vi "Services.Compile.vi"(8 "error in (no error)":errorcluster, 11 "Section Ref in":T4 format="%.0x") -> (0 "error out":errorcluster, 2 "Settings":T1[](array[typedef]) {"Signal.Cmd.Refs"."Signal Refs" format="%.0x"; "Signal.Cmd.Info"."Signals"."Byte Order" items=["Little Endian", "Big Endian"]; "Signal.Cmd.Info"."Signals"."Data Type" items=["Signed", "Unsigned", "IEEE Float"]; "Settings.Refs"."Signal Refs" format="%.0x"; "Signal.Resp.Refs"."Signal Refs" format="%.0x"; "Signal.Resp.Info"."Signals"."Byte Order" items=["Little Endian", "Big Endian"]; "Signal.Resp.Info"."Signals"."Data Type" items=["Signed", "Unsigned", "IEEE Float"]; "Trigger.Refs"."Signal Refs" format="%.0x"; "Status.Refs"."Signal Refs" format="%.0x"}, 3 "Section Ref out":T4 format="%.0x")   [LabVIEW 2019, in "Diagnostics Addon System Explorer.lvlib"]
uses:
  Diagnostics Addon System Explorer.lvlib
  <vilib>/NI VeriStand/Custom Device Tools/Custom Device Utility Library/Custom Device Utility Library.lvlib
  Types/Frame.Ref.ctl
  Types/FG.Action.ctl
  <vilib>/NI VeriStand/Custom Device API/Custom Device Item Ref.ctl
  <vilib>/NI VeriStand/Custom Device API/Custom Device API.lvlib
  Addon Shared/Types/Signal.ctl
  Addon Shared/Diagnostics Addon Shared.lvlib
  Addon Shared/Types/Frame.Compile.ctl
  Addon Shared/Types/Type.ctl
  Types/Service.Export.ctl
  <vilib>/NI VeriStand/Custom Device Tools/Custom Device Utility Library/NI VeriStand - Search for Item by GUID.vi
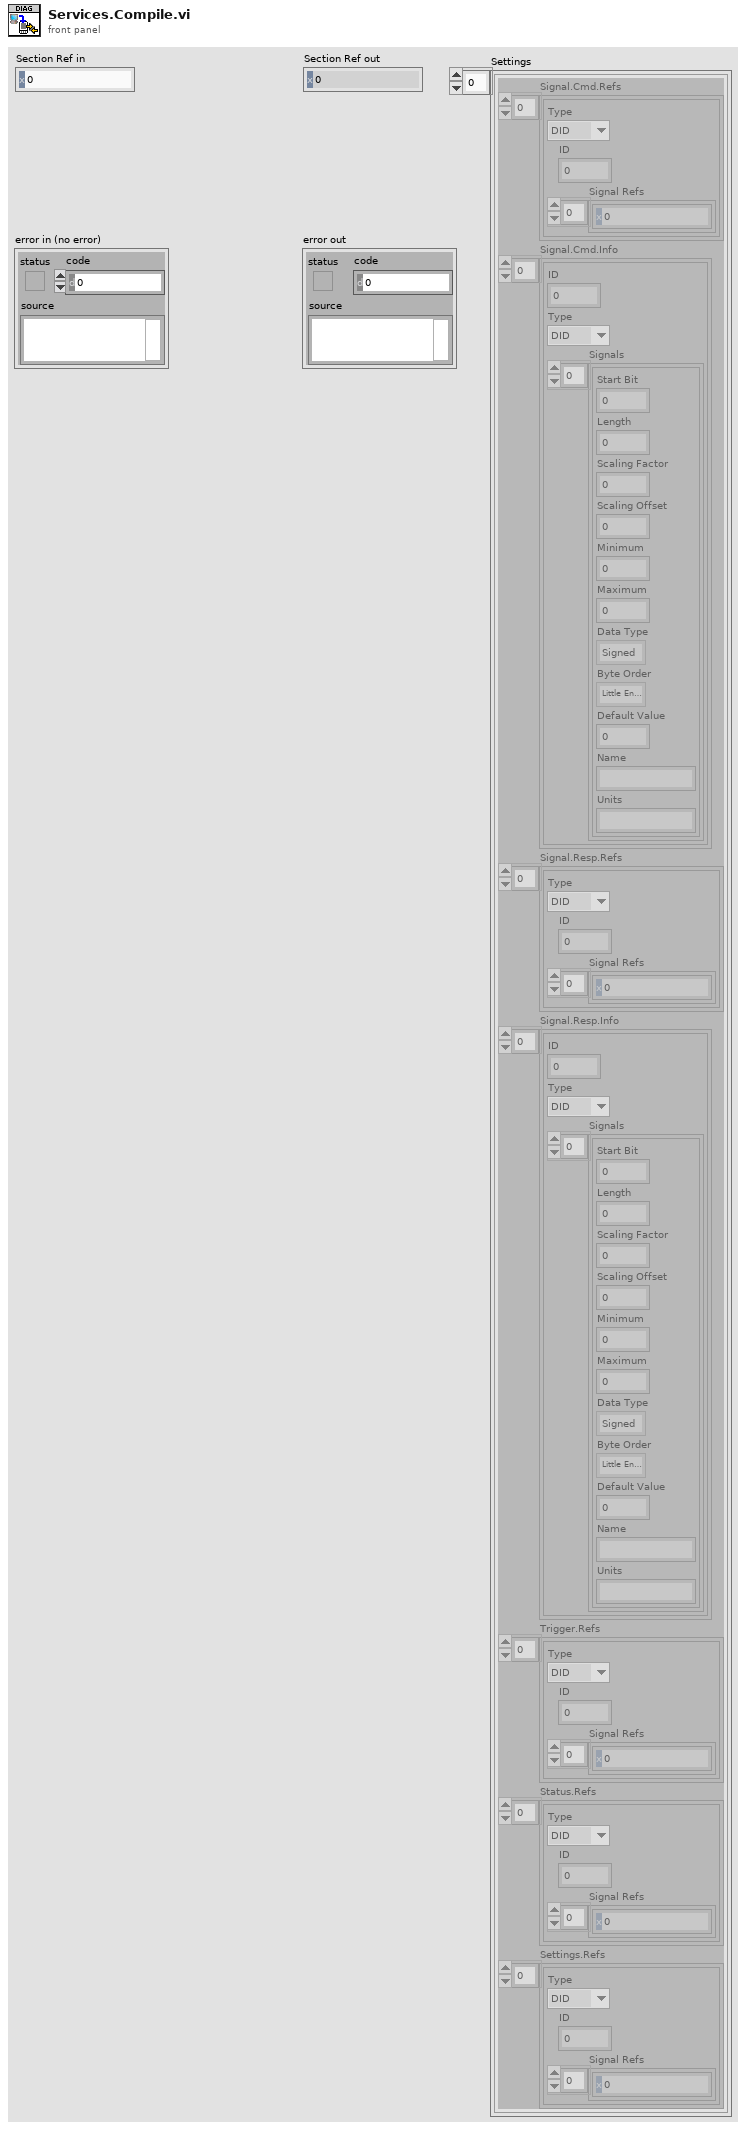
[diagram p1: front panel]
types:
  T1 = typedef "Diagnostics Addon System Explorer.lvlib/Service.Export.ctl" = cluster{"Signal.Cmd.Refs":T2[], "Signal.Cmd.Info":T5[], "Signal.Resp.Refs":T2[], "Signal.Resp.Info":T5[], "Trigger.Refs":T2[], "Status.Refs":T2[], "Settings.Refs":T2[]}
  T2 = typedef "Diagnostics Addon System Explorer.lvlib/Frame.Ref.ctl" = cluster{"Type":T3, "ID":u32, "Signal Refs":T4[]}
  T3 = typedef "Diagnostics Addon Shared.lvlib/Type.ctl" = enum16{"DID", "CDID", "PID", "CPID", "Read Memory", "Write Memory", "IO Control", "Routine Start", "Routine Request", "Routine Stop", "User Defined", "DTC Control", "Clear DTCs", "Read DTCs", "Start DTCs", "DTC Change Count", "Tester Present", "Unlock ECU", "Reset ECU", "Diag Session Control", "Communication Control", "DPID Control", "Poll Control", "Diag Comm Port Control"}
  T4 = typedef "Custom Device API.lvlib/Custom Device Item Ref.ctl" = u64
  T5 = typedef "Diagnostics Addon Shared.lvlib/Frame.Compile.ctl" = cluster{"ID":u32, "Type":T3, "Signals":T6[]}
  T6 = typedef "Diagnostics Addon Shared.lvlib/Signal.ctl" = cluster{"Start Bit":u32, "Length":u32, "Scaling Factor":dbl, "Scaling Offset":dbl, "Minimum":dbl, "Maximum":dbl, "Data Type":u32, "Byte Order":u32, "Default Value":dbl, "Name":string, "Units":string}
  T7 = typedef "Diagnostics Addon System Explorer.lvlib/FG.Action.ctl" = enum16{"Get", "Set"}
  T8 = typedef "Diagnostics Addon Shared.lvlib/CAN.ctl" = cluster{"Interface":T9, "Baud Rate":u64, "Diagnostic Protocol":T10, "Transport Protocol":T11, "Transmit ID":u32, "Receive ID":u32, "Transmit Extension":u8, "Receive Extension":u8, "Receive UUDT ID":u32, "Enable Stream":bool, "VW TP Channel ID":u32, "Fill Frame":bool, "Fill Byte":u8, "Termination":bool, "LIN Cluster":refnum<k21>, "NAD":u8, "IO Mode":u32, "Max DLC":u16, "FD Baud Rate":u64, "Timeout":u32, "FD ISO Mode":u32, "DoIP Address":string, "DoIP Source Address":u16, "DoIP Dynamic Port":bool, "DoIP Version":u16}
  T9 = typedef "Diagnostics Addon Shared.lvlib/CAN.Interface.ctl" = string
  T10 = typedef "Diagnostics Addon Shared.lvlib/Protocol.ctl" = enum16{"GMLAN", "KWP-2000", "UDS", "User-Defined"}
  T11 = typedef "Diagnostics Addon Shared.lvlib/Transport.ctl" = enum16{"ISO TP - Normal Mode", "ISO TP - Mixed Mode", "VW TP 2.0", "Diagnostics on IP", "ISO TP LIN"}
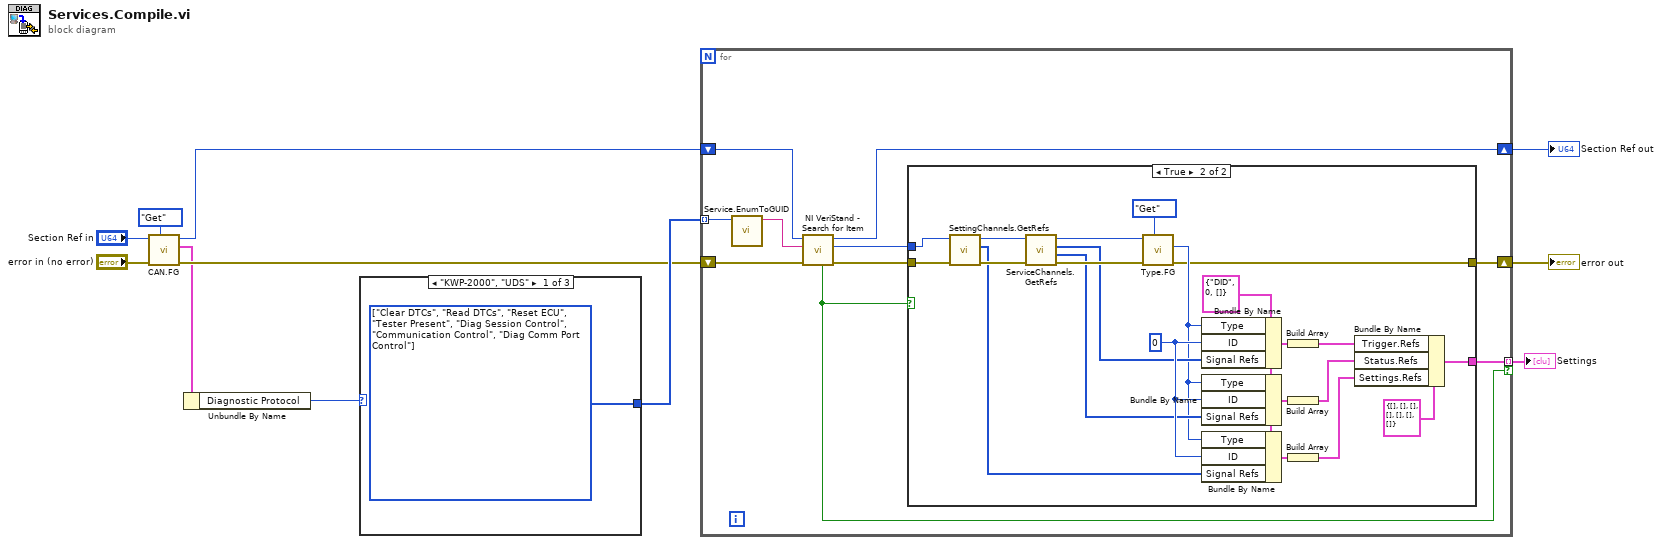
[diagram p0: block diagram]
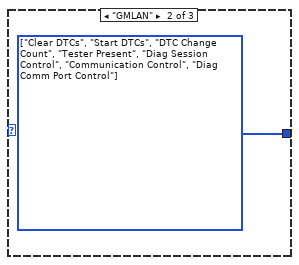
[diagram p2: hidden frame]
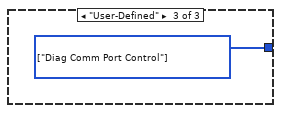
[diagram p3: hidden frame]
diagram:
  n1 = call "CAN.FG.vi"("Action"=FG.Action."Get", "error in (no error)"="error in (no error)", "Device Item Ref in"="Section Ref in") -> ("error out"=w5:errorcluster, "Diagnostics Basic Configuration"=w2:T8, "Device Item Ref out"=w3:T4)  [unwired: 6 in]
  n2 = Unbundle By Name(w2) -> ("Diagnostic Protocol"=w1:T10)
  n3 = case shown="\"KWP-2000\", \"UDS\"" w1 {
    tunnel: [w12 w13 w14] -> w8
    frame "KWP-2000", "UDS" {
      w12 = T3[] [enum."Clear DTCs", enum."Read DTCs", enum."Reset ECU", enum."Tester Present", enum."Diag Session Control", enum."Communication Control", enum."Diag Comm Port Control"] items=["DID", "CDID", "PID", "CPID", "Read Memory", "Write Memory", "IO Control", "Routine Start", "Routine Request", "Routine Stop", "User Defined", "DTC Control", "Clear DTCs", "Read DTCs", "Start DTCs", "DTC Change Count", "Tester Present", "Unlock ECU", "Reset ECU", "Diag Session Control", "Communication Control", "DPID Control", "Poll Control", "Diag Comm Port Control"]
    }
    frame "GMLAN" {
      w13 = T3[] [enum."Clear DTCs", enum."Start DTCs", enum."DTC Change Count", enum."Tester Present", enum."Diag Session Control", enum."Communication Control", enum."Diag Comm Port Control"] items=["DID", "CDID", "PID", "CPID", "Read Memory", "Write Memory", "IO Control", "Routine Start", "Routine Request", "Routine Stop", "User Defined", "DTC Control", "Clear DTCs", "Read DTCs", "Start DTCs", "DTC Change Count", "Tester Present", "Unlock ECU", "Reset ECU", "Diag Session Control", "Communication Control", "DPID Control", "Poll Control", "Diag Comm Port Control"]
    }
    frame "User-Defined" {
      w14 = T3[] [enum."Diag Comm Port Control"] items=["DID", "CDID", "PID", "CPID", "Read Memory", "Write Memory", "IO Control", "Routine Start", "Routine Request", "Routine Stop", "User Defined", "DTC Control", "Clear DTCs", "Read DTCs", "Start DTCs", "DTC Change Count", "Tester Present", "Unlock ECU", "Reset ECU", "Diag Session Control", "Communication Control", "DPID Control", "Poll Control", "Diag Comm Port Control"]
    }
  }
  n4 = for {
    tunnel: [w18] -> w9 mode=indexing if=w17
    shift-right: [w20] -> w11
    shift-left: w3 -> [w22]
    shift-right: [w19] -> w10
    shift-left: w5 -> [w21]
    tunnel: w8 -> [w15] mode=indexing
    n5 = call "Service.EnumToGUID.vi"("Type"=w15) -> ("GUID"=w16:string)  [unwired: 10 in]
    n6 = call-poly <vilib>:"NI VeriStand - Search for Item.vi"("error in"=w21, "Item GUID"=w16, "Section Ref in"=w22) -> ("error out"=w23:errorcluster, "Item Ref"=w24:T4, "Section Ref out"=w20:T4, "Found"=w17:bool)  [unwired: 5 in]
    n7 = case shown="True" w17 {
      tunnel: [w25 w26] -> w19
      tunnel: w24 -> [_ w39]
      tunnel: w23 -> [w25 w41]
      tunnel: [_ w45] -> w18
      frame False {
      }
      frame True {
        w35 = 0
        w34 = T2 {"Type"=enum."DID", "ID"=0, "Signal Refs"=[]} ("cluster")
        n8 = call "SettingChannels.GetRefs.vi"("error in (no error)"=w41, "Item Ref in"=w39) -> ("error out"=w44:errorcluster, "Settings"=w31:T4[], "Section Ref out"=w43:T4)  [unwired: 7 in]
        n9 = call "ServiceChannels.GetRefs.vi"("error in (no error)"=w44, "Item Ref in"=w43) -> ("error out"=w42:errorcluster, "Status"=w32:T4[], "Trigger"=w33:T4[], "Section Ref out"=w40:T4)  [unwired: 6 in]
        n10 = call "Type.FG.vi"("Action"=FG.Action."Get", "error in (no error)"=w42, "Device Item Ref in"=w40) -> ("error out"=w26:errorcluster, "Type"=w27:T3)  [unwired: 6 in, 1 out]
        n11 = Bundle By Name(cluster=w34, "Type"=w27, "ID"=w35, "Signal Refs"=w33) -> (w38:T2)
        n12 = Bundle By Name(cluster=w34, "Type"=w27, "ID"=w35, "Signal Refs"=w32) -> (w37:T2)
        n13 = Bundle By Name(cluster=w34, "Type"=w27, "ID"=w35, "Signal Refs"=w31) -> (w36:T2)
        n14 = Build Array(w38) -> (w30:T2[])
        n15 = Build Array(w37) -> (w29:T2[])
        n16 = Build Array(w36) -> (w28:T2[])
        n17 = Bundle By Name(cluster=T1 {"Signal.Cmd.Refs"=[], "Signal.Cmd.Info"=[], "Signal.Resp.Refs"=[], "Signal.Resp.Info"=[], "Trigger.Refs"=[], "Status.Refs"=[], "Settings.Refs"=[]}, "Trigger.Refs"=w30, "Status.Refs"=w29, "Settings.Refs"=w28) -> (w45:T1)
      }
    }
  }
  "Section Ref out" <- w11
  "error out" <- w10
  "Settings" <- w9
